vi "folder_exist.vi"(2 "error in (no error)":errorcluster, 3 "TestDay":u16(ring) items=["Day-0", "Day-1", "Day-2", "Day-3", "Day-4", "Day-5", "Day-6", "Day-7", "Day-8", "Day-9"], 4 "path":path) -> (0 "error out":errorcluster, 1 "new_folder":path)   [LabVIEW 2012]
uses:
  Global_var.vi
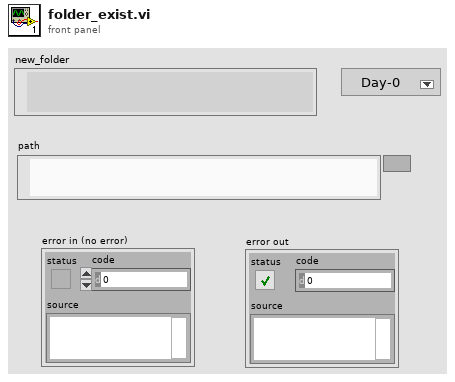
[diagram p1: front panel]
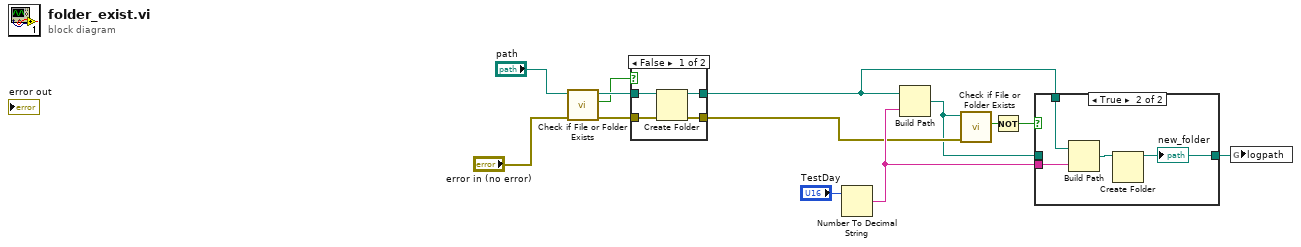
[diagram p0: block diagram]
diagram:
  n1 = call <vilib>:"Check if File or Folder Exists.vi"("error in (no error)"="error in (no error)", "path"="path") -> ("error out"=w10:errorcluster, "file or folder exists?"=w11:bool, "dup path"=w12:path)  [unwired: 7 in]
  n2 = case shown="False" w11 {
    tunnel: w12 -> [w17 w19]
    tunnel: w10 -> [w16 w18]
    tunnel: [w15 w19] -> w6
    tunnel: [w14 w18] -> w5
    frame False {
      n3 = Create Folder(path (use dialog)=w17, error in=w16) -> (created path=w15:path, error out=w14:errorcluster)  [unwired: 1 in, 1 out]
    }
    frame True {
    }
  }
  n4 = Number To Decimal String(number="TestDay") -> (decimal integer string=w13:string)  [unwired: 1 in]
  n5 = Build Path(base path=w6, name or relative path=w13) -> (appended path=w1:path)
  n6 = call <vilib>:"Check if File or Folder Exists.vi"("error in (no error)"=w5, "path"=w1) -> ("file or folder exists?"=w7:bool)  [unwired: 7 in, 2 out]
  n7 = Not(x=w7) -> (.not. x?=w3:bool)
  n8 = case shown="True" w3 {
    tunnel: w13 -> [_ w24]
    tunnel: w6 -> [_ w22]
    tunnel: [w20 w21] -> w2
    tunnel: w1 -> [w20 _]
    frame False {
    }
    frame True {
      n9 = Build Path(base path=w22, name or relative path=w24) -> (appended path=w23:path)
      n10 = Create Folder(path (use dialog)=w23) -> (created path=w21:path)  [unwired: 2 in, 2 out]
      "new_folder" <- w21
    }
  }
  n11 = global write "Global_var.vi" "logpath"(w2) -> ()
